vi "CheckForEOL.vi"(11 "REPL":string) -> (3 "Complete?":bool)   [LabVIEW 2020]
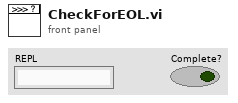
[diagram p1: front panel]
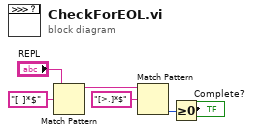
[diagram p0: block diagram]
diagram:
  n1 = Match Pattern(string="REPL", regular expression="[ ]*$") -> (before substring=w3:string)  [unwired: 1 in, 3 out]
  n2 = Match Pattern(string=w3, regular expression="[>.]*$") -> (offset past match=w4:i32)  [unwired: 1 in, 3 out]
  n3 = Greater Or Equal To 0?(x=w4) -> (x >= 0?=→"Complete?":bool)
